vi "发送消息.vi"(7 "强制优先":bool, 8 "错误输入（无错误）":errorcluster, 9 "数据":variant, 10 "消息":string, 11 "输入队列":refnum<queue>) -> (0 "错误输出":errorcluster, 3 "输出队列":refnum<queue>)   [LabVIEW 2021, in "QueueLib.lvlib"]
uses:
  QueueLib.lvlib
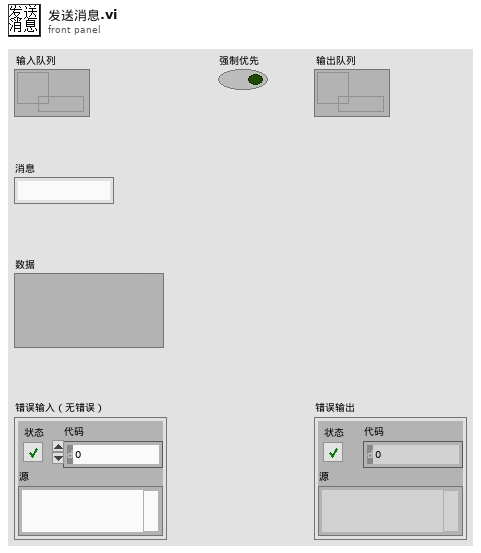
[diagram p1: front panel]
types:
  T1 = typedef "QueueLib.lvlib/数据类型.ctl" = cluster{"消息":string, "数据":variant}
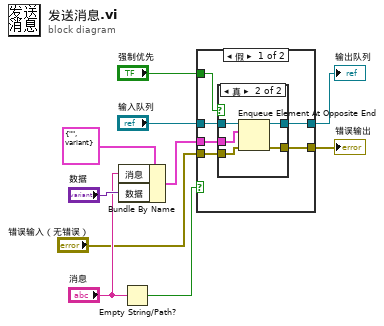
[diagram p0: block diagram]
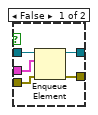
[diagram p2: hidden frame]
diagram:
  n1 = Bundle By Name(cluster=T1 {"消息"="", "数据"=variant} ("数据类型"), "消息"="消息", "数据"="数据") -> (w6:T1)
  n2 = Empty String/Path?(string/path="消息") -> (empty?=w10:bool)
  n3 = case shown="假" w10 {
    tunnel: "输入队列" -> [w16 w27]
    tunnel: w6 -> [w15 _]
    tunnel: "错误输入（无错误）" -> [w14 w28]
    tunnel: "强制优先" -> [w13 _]
    tunnel: [w12 w28] -> w3
    tunnel: [w11 w27] -> w2
    frame False {
      n4 = case shown="真" w13 {
        tunnel: w16 -> [w21 w26]
        tunnel: w15 -> [w20 w24]
        tunnel: w14 -> [w19 w23]
        tunnel: [w18 w22] -> w12
        tunnel: [w17 w25] -> w11
        frame False {
          n5 = Enqueue Element(queue=w21, element=w20, error in (no error)=w19) -> (queue out=w17:refnum<queue>, error out=w18:errorcluster)  [unwired: 1 in, 1 out]
        }
        frame True {
          n6 = Enqueue Element At Opposite End(queue=w26, element=w24, error in (no error)=w23) -> (queue out=w25:refnum<queue>, error out=w22:errorcluster)  [unwired: 1 in, 1 out]
        }
      }
    }
    frame True {
    }
  }
  "错误输出" <- w3
  "输出队列" <- w2
